vi "CopyAttributes.vi"(8 "error in (no error)":errorcluster, 10 "Attributes":variant, 11 "BrowerComponent in":refnum<class "BrowerComponent.lvclass">) -> (0 "error out":errorcluster, 3 "BrowerComponent out":refnum<class "BrowerComponent.lvclass">)   [LabVIEW 2015]
uses:
  BrowerComponent.lvclass
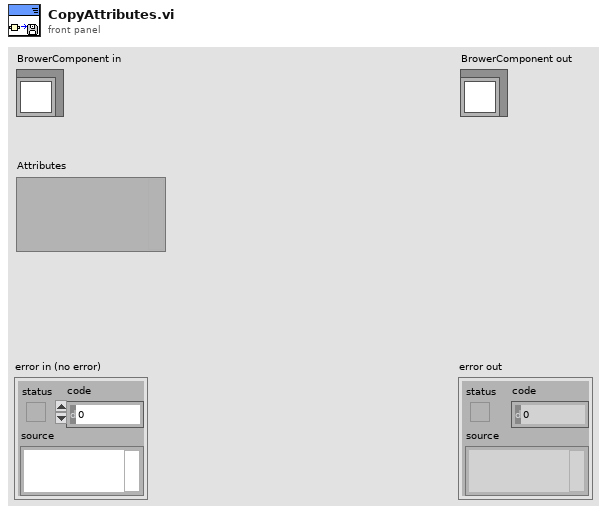
[diagram p1: front panel]
types:
  T1 = typedef "BrowerComponent.lvclass/ObjectAttributes.ctl" = cluster{"ComponentID":string, "SymbolIndex":i32, "ComponentName":string, "PartsOfComponent_dict":variant}
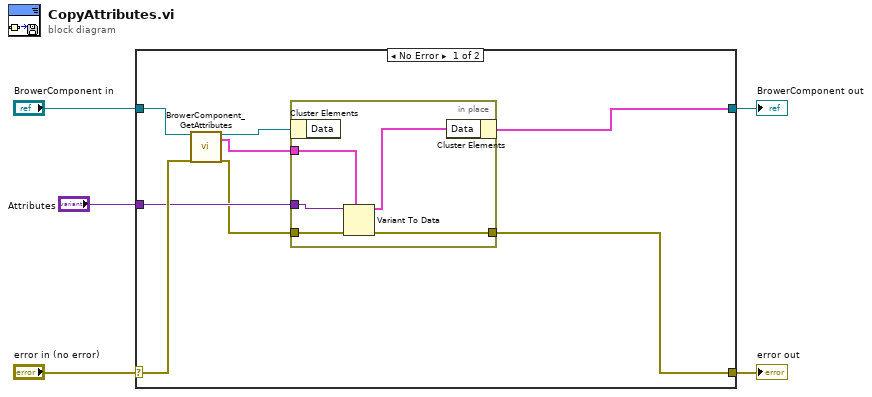
[diagram p0: block diagram]
diagram:
  n1 = case shown="No Error" "error in (no error)" {
    selector: "error in (no error)" -> [w12 w20]
    tunnel: [w6 w20] -> w4
    tunnel: [w9 w19] -> w2
    tunnel: "BrowerComponent in" -> [w13 w19]
    tunnel: "Attributes" -> [w8 _]
    frame No Error {
      n2 = call "BrowerComponent_GetAttributes.vi"("reference in"=w13, "error in (no error)"=w12) -> ("reference out"=w11:refnum<class "BrowerComponent.lvclass">, "Data"=w10:T1, "error out"=w7:errorcluster)  [unwired: 14 in, 1 out]
      n3 = in-place {
        in-place-border: w10 -> [w17]
        in-place-border: w8 -> [w18]
        in-place-border: w7 -> [w16]
        in-place-border: [w15] -> w6
        n4 = in-place-cluster #1(w11) -> ()  [unwired: 1 out]
        n5 = Variant To Data(error in=w16, type=w17, Variant=w18) -> (data=w14:T1, error out=w15:errorcluster)
        n6 = in-place-cluster #1("Data"=w14) -> (w9:cluster{})
      }
    }
    frame Error {
    }
  }
  "error out" <- w4
  "BrowerComponent out" <- w2
